vi "WINDOWS.AUTO SIZE.vi"(4 "Error In":errorcluster, 6 "TAB.AutoAjuste":refnum<vi>, 7 "This VI":refnum<vi>) -> (0 "Error Out":errorcluster)   [LabVIEW 2019]
doc: "<B>NOMBRE VI:</B>\nWINDOWS.AUTO SIZE.vi\n\n<B>DESCRIPCION:</B>\nEste VI ajusta el tamaño front panel al tamaño de un control TAB. De forma que si este control TAB cambia de tamaño por el diseño de nuestra aplicación la ventana front panel también cambiara de tamaño y se ajustara al mismo tamaño que control TAB. Así evitamos tener que ajustarla cada vez que cambiemos algo.\n\n<B>ENTRADA:</B>\n>______This VI______<\nRefNum de la ventana front panel que deseamos modificar.\n\n>______TAB.AutoAjuste______<\nRefNum del control TAB que nos servirá como referencia para ajustar el tamaño de la ventana front panel\n\n>______Error In______<\nCluster de errores.\n\n<B>SALIDA:</B>\n>______Error Out\nEste programa no debería de modificar el cluster de error ya que he deshabilitado los errores de los Property Nodes para evitar interrupciones en el programa..\n\n<B>FUNCIONAMIENTO:</B>\nLo primero es ocultar Label, Tag y pestañas en el control TAB, después adquirimos el tamaño (Bounds) y la posición (Position) de este control en función del front panel.\nAdquirir el tamaño y posición que ocupa el front panel (FP.PanelBounds) y lo modificaremos para que tenga el mismo tamaño que el control TAB. Además colocaremos el origen del front panel a la posición que tiene el control TAB.\n\n<B>NOTA PARA EL PROBRAMADOR:</B>\nComo algunas veces nos olvidamos:\nPara crear las referencias del VI y del control, nos vamos a Application Control (La mano con la bandeja) y pulsamos sobre VI Server Referente, de esta forma obtendremos la referencia de nuestro VI, ahora podemos copiarlo y pulsamos con el boton derecho sobre esta copia, se abre un menú emergente y seleccionamos Link To y elegimos el control Tab que nos sirve de referencia.\nAdemas tenemos que ocultar las Page Label Displays del control TAB y las Scroll bar de nuestro VI."
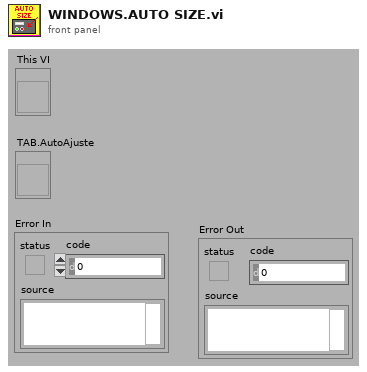
[diagram p1: front panel]
types:
  T1 = enum16{"Always On", "Always Off", "Off While Running"}
  T2 = typedef "LVPositionTypeDef.ctl" = cluster{"Left":i32, "Top":i32}
  T3 = typedef "LVBoundsTypeDef.ctl" = cluster{"Width":u32, "Height":u32}
  T4 = typedef "LVRectTypeDef.ctl" = cluster{"Left":i16, "Top":i16, "Right":i16, "Bottom":i16}
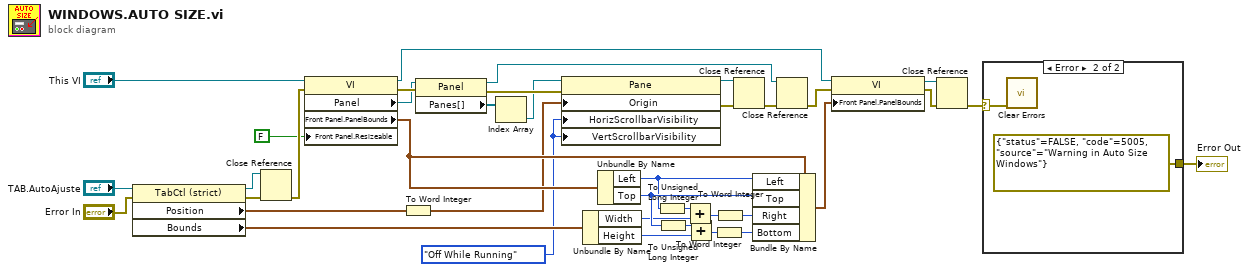
[diagram p0: block diagram]
diagram:
  w11 = T1."Off While Running" ("Vertical Scrollbar Visibility")
  n1 = property class="TabCtl (strict)"(reference="TAB.AutoAjuste", error in="Error In") -> (reference out=w14:refnum<vi>, error out=w13:errorcluster, "Position"=w29:T2, "Bounds"=w30:T3)
  n2 = Close Reference(reference=w14, error in (no error)=w13) -> (error out=w15:errorcluster)
  n3 = property class="VI"(reference="This VI", error in=w15, "Front Panel.Resizeable"=FALSE ("Front Panel Window:Resizable")) -> (reference out=w25:refnum<vi>, error out=w17:errorcluster, "Panel"=w16:refnum<vi>, "Front Panel.PanelBounds"=w31:T4)
  n4 = To Word Integer(number=w29) -> (16bit integer=w2:cluster{"Left":i16, "Top":i16})
  n5 = property class="Panel"(reference=w16, error in=w17) -> (reference out=w24:refnum<vi>, error out=w20:errorcluster, "Panes[]"=w18:refnum<vi>[])
  n6 = Index Array(array=w18) -> (element=w19:refnum<vi>)  [unwired: 1 in]
  n7 = property class="Pane"(reference=w19, error in=w20, "Origin"=w2, "HorizScrollbarVisibility"=w11, "VertScrollbarVisibility"=w11) -> (reference out=w23:refnum<vi>, error out=w21:errorcluster)
  n8 = Unbundle By Name(w30) -> ("Width"=w33:u32, "Height"=w36:u32)
  n9 = Unbundle By Name(w31) -> ("Left"=w32:i16, "Top"=w35:i16)
  n10 = To Unsigned Long Integer(number=w32) -> (unsigned 32bit integer=w8:u32)
  n11 = To Unsigned Long Integer(number=w35) -> (unsigned 32bit integer=w7:u32)
  n12 = Add(x=w8, y=w33) -> (x+y=w34:u32)
  n13 = Add(x=w7, y=w36) -> (x+y=w37:u32)
  n14 = To Word Integer(number=w37) -> (16bit integer=w5:i16)
  n15 = To Word Integer(number=w34) -> (16bit integer=w6:i16)
  n16 = Close Reference(reference=w23, error in (no error)=w21) -> (error out=w22:errorcluster)
  n17 = Bundle By Name(cluster=w31, "Left"=w32, "Top"=w35, "Right"=w6, "Bottom"=w5) -> (w38:T4)
  n18 = Close Reference(reference=w24, error in (no error)=w22) -> (error out=w26:errorcluster)
  n19 = property class="VI"(reference=w25, error in=w26, "Front Panel.PanelBounds"=w38) -> (reference out=w28:refnum<vi>, error out=w27:errorcluster)
  n20 = Close Reference(reference=w28, error in (no error)=w27) -> (error out=w4:errorcluster)
  n21 = case shown="Error" w4 {
    selector: w4 -> [w39 w40]
    tunnel: [w39 errorcluster {"status"=FALSE, "code"=5005, "source"="Warning in Auto Size Windows"} ("error in (no error)")] -> w3
    frame No Error {
    }
    frame Error {
      n22 = call <vilib>:"Clear Errors.vi"("error in (no error)"=w40) -> ()  [unwired: 5 in, 2 out]
    }
  }
  "Error Out" <- w3
